vi "Read.vi"(11 "ConfigElementValue in":refnum<class "ConfigElementValue.lvclass">) -> (2 "Config Element":refnum<class "Config Element.lvclass">)   [LabVIEW 2020, in "Volatus.lvlib" / "ConfigElementValue.lvclass"]
uses:
  ConfigElementValue.lvclass
  ConfigElementValue.lvclass/ConfigElementValue.ctl
  lv-cdm/CDM-Config/Config Element/Config Element.lvclass
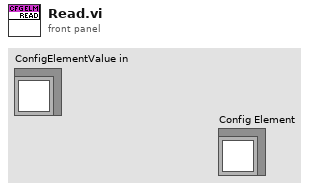
[diagram p1: front panel]
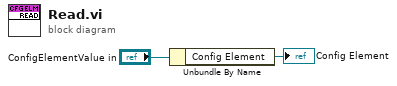
[diagram p0: block diagram]
diagram:
  n1 = Unbundle By Name("ConfigElementValue in") -> ("Config Element"=→"Config Element":refnum<class "Config Element.lvclass">)
